vi "Main.vi"(8 "error in (no error)":errorcluster, 11 "ExampleClassDScaffold in":refnum<class "ExampleClassDScaffold.lvclass">) -> (0 "error out":errorcluster, 3 "ExampleClassDScaffold out":refnum<class "ExampleClassDScaffold.lvclass">)   [LabVIEW 2012, in "ExampleClassDScaffold.lvclass"]
doc: "Main VI of the component. This should contain the GUI of your component and be called when creating an executable."
uses:
  ExampleClassDScaffold.lvclass
  <vilib>/Distrio/Murmex/InitialiseMessage/InitialiseMessage.lvclass
  <vilib>/Distrio/Murmex/Murmex/Set configure at initialise.vi
  <vilib>/Distrio/Murmex/Murmex/Set VI reference.vi
  <vilib>/Distrio/Murmex/Murmex/Set log reference.vi
  <vilib>/Distrio/Murmex/Murmex/Get component name.vi
  <vilib>/Distrio/Murmex/Murmex/Get ID.vi
  <vilib>/Distrio/Murmex/Murmex/Set relay start stop to observers.vi
  <vilib>/Distrio/Murmex/Murmex/Murmex.lvclass
panel:
  out "log":string
  out "component":string
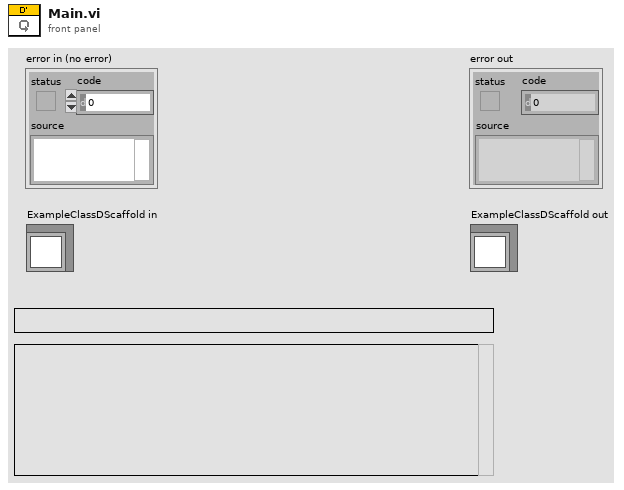
[diagram p1: front panel]
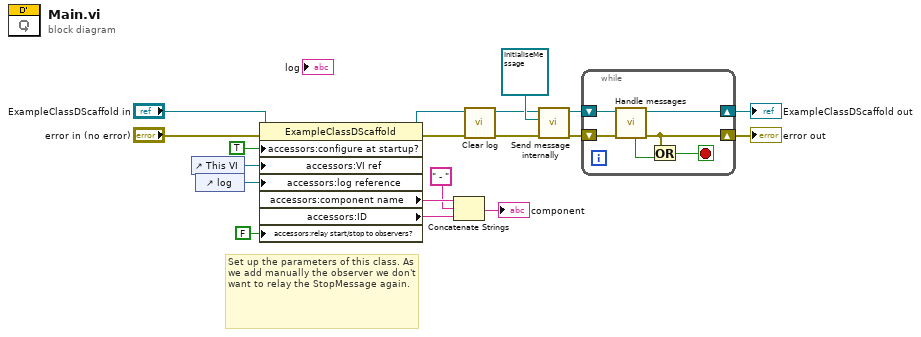
[diagram p0: block diagram]
diagram:
  # "Set up the parameters of this class. As we add manually the observer we don't want to relay the StopMessage again."
  n1 = control-ref of="This VI"() -> (w11:refnum<vi>)
  n2 = control-ref of="log"() -> (w10:refnum<vi>)
  n3 = property class="ExampleClassDScaffold"(reference="ExampleClassDScaffold in", error in="error in (no error)", "accessors:configure at startup?"=TRUE ("configure at startup?"), "accessors:VI ref"=w11, "accessors:log reference"=w10, "accessors:relay start/stop to observers?"=FALSE ("relay start/stop to observers?")) -> (reference out=w7:refnum<class "ExampleClassDScaffold.lvclass">, error out=w15:errorcluster, "accessors:component name"=w5:string, "accessors:ID"=w4:string)
  n4 = Concatenate Strings(w5, " - " ("string"), w4) -> (→"component":string)
  n5 = call <vilib>:"Clear log.vi"("error in (no error)"=w15, "MurmexBase in"=w7) -> ("error out"=w8:errorcluster, "MurmexBase out"=w6:refnum<class "ExampleClassDScaffold.lvclass">)  [unwired: 8 in]
  n6 = call <vilib>:"Send message internally.vi"("error in (no error)"=w8, "Message"=refnum<class "InitialiseMessage.lvclass"> refnum ("Distrio Murmex 1.5:InitialiseMessage"), "Murmex in"=w6) -> ("error out"=w14:errorcluster, "Murmex out"=w16:refnum<class "ExampleClassDScaffold.lvclass">)  [unwired: 7 in]
  n7 = while {
    shift-right: [w22] -> w19
    shift-left: w14 -> [w24]
    shift-right: [w25] -> w18
    shift-left: w16 -> [w23]
    stop <- w20 stop-if-true
    n8 = call <vilib>:"Handle messages.vi"("error in (no error)"=w24, "Murmex in"=w23) -> ("error out"=w22:errorcluster, "Murmex out"=w25:refnum<class "ExampleClassDScaffold.lvclass">, "terminated?"=w21:bool)  [unwired: 7 in]
    n9 = Or(x=w22, y=w21) -> (x .or. y?=w20:bool)
  }
  "error out" <- w19
  "ExampleClassDScaffold out" <- w18
